vi "Mobility-Vt-Used Pts_Saturation.vi"(5 "Width":dbl, 6 "Dielectric Const":dbl, 7 "Length":dbl, 9 "Dielectric (d)":dbl, 10 "Sat Id Used":dbl[](array[numeric]), 11 "Vg Used":dbl[](array[numeric])) -> (1 "Capacitance":dbl, 2 "Vt":dbl, 3 "Mobility":dbl)   [LabVIEW 2012]
uses:
  <vilib>/Analysis/NI_AALPro.lvlib
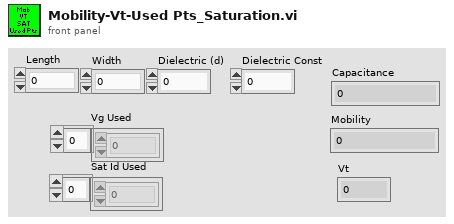
[diagram p1: front panel]
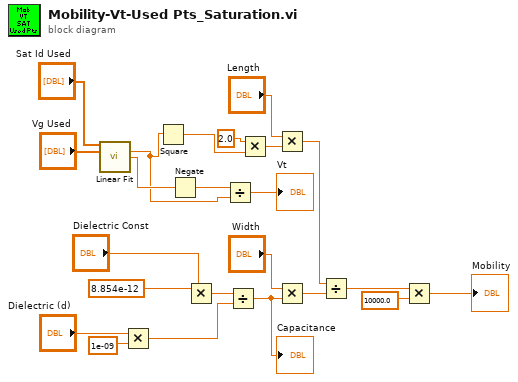
[diagram p0: block diagram]
diagram:
  n1 = call <vilib>:"Linear Fit.vi"("Y"="Sat Id Used", "X"="Vg Used") -> ("slope"=w3:dbl, "intercept"=w4:dbl)  [unwired: 9 in, 3 out]
  n2 = Multiply(x="Dielectric (d)", y=1e-09) -> (x*y=w22:dbl)
  n3 = Square(x=w3) -> (x^2=w2:dbl)
  n4 = Negate(x=w4) -> (-x=w6:dbl)
  n5 = Multiply(x=8.854e-12, y="Dielectric Const") -> (x*y=w23:dbl)
  n6 = Divide(x=w6, y=w3) -> (x/y=→"Vt":dbl)
  n7 = Divide(x=w23, y=w22) -> (x/y=w5:dbl)
  "Capacitance" <- w5
  n8 = Multiply(x=2.0, y=w2) -> (x*y=w16:dbl)
  n9 = Multiply(x="Length", y=w16) -> (x*y=w15:dbl)
  n10 = Multiply(x="Width", y=w5) -> (x*y=w14:dbl)
  n11 = Divide(x=w15, y=w14) -> (x/y=w12:dbl)
  n12 = Multiply(x=w12, y=10000.0) -> (x*y=→"Mobility":dbl)
